vi "PositionCountTest.vi"() -> ()   [LabVIEW 2015]
uses:
  QuadEnc/QuadEnc.lvlib
panel:
  out "RevPosition 2":i32
  out "AbsPosition 2":i32
  in  "number of iterations":i32=20
  in  "spoofed tick rate":u32=20
  in  "spoofed ticks per rev":u32=10
  out "RevPosition":i32=999
  out "AbsPosition":i32=1999
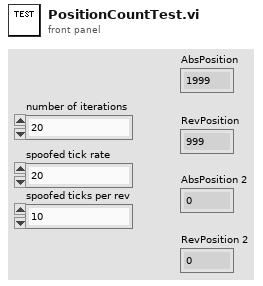
[diagram p1: front panel]
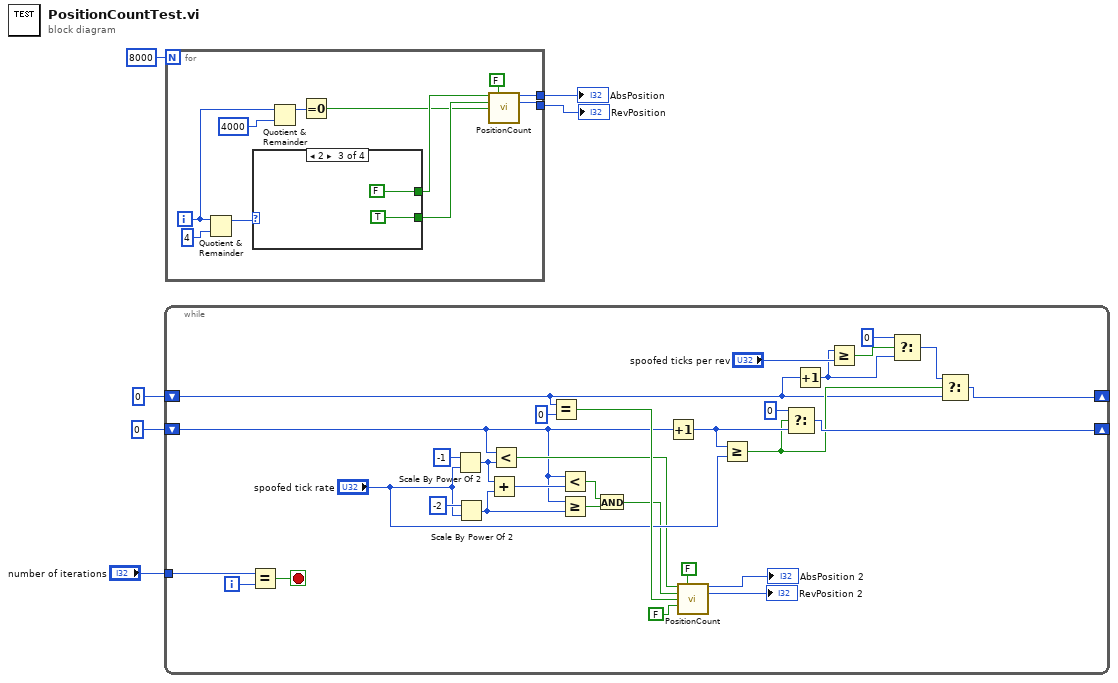
[diagram p0: block diagram]
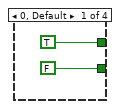
[diagram p2: hidden frame]
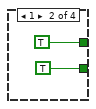
[diagram p3: hidden frame]
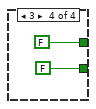
[diagram p4: hidden frame]
diagram:
  n1 = while {
    shift-right: [w26] -> _
    shift-left: u32 0 -> [w11]
    shift-right: [w25] -> _
    shift-left: u32 0 -> [w10]
    tunnel: "number of iterations" -> [w18]
    i -> [w16]
    stop <- w24 stop-if-true
    n2 = Equal?(x=w18, y=w16) -> (x = y?=w24:bool)
    n3 = Scale By Power Of 2(n=i16 -1, x="spoofed tick rate") -> (x*2^n=w34:u32)
    n4 = Scale By Power Of 2(n=i16 -2, x="spoofed tick rate") -> (x*2^n=w33:u32)
    n5 = Add(x=w34, y=w33) -> (x+y=w32:u32)
    n6 = Less?(x=w11, y=w34) -> (x < y?=w13:bool)
    n7 = Equal?(x=w10, y=u32 0) -> (x = y?=w19:bool)
    n8 = Less?(x=w11, y=w32) -> (x < y?=w31:bool)
    n9 = Greater Or Equal?(x=w11, y=w33) -> (x >= y?=w30:bool)
    n10 = And(x=w31, y=w30) -> (x .and. y?=w14:bool)
    n11 = Increment(x=w11) -> (x+1=w27:u32)
    n12 = call "PositionCount.vi"("A"=w13, "ReversePolarity"=FALSE, "B"=w14, "Z"=w19, "reset"=FALSE) -> ("AbsPosition"=→"AbsPosition 2":i32, "RevPosition"=→"RevPosition 2":i32)  [unwired: 8 in, 1 out]
    n13 = Greater Or Equal?(x=w27, y="spoofed tick rate") -> (x >= y?=w12:bool)
    n14 = Select(t=u32 0, s=w12, f=w27) -> (s? t:f=w26:u32)
    n15 = Increment(x=w10) -> (x+1=w8:u32)
    n16 = Greater Or Equal?(x=w8, y="spoofed ticks per rev") -> (x >= y?=w9:bool)
    n17 = Select(t=u32 0 ("s? t:f"), s=w9, f=w8) -> (s? t:f=w7:u32)
    n18 = Select(t=w7, s=w12, f=w10) -> (s? t:f=w25:u32)
  }
  n19 = for {
    N: 8000 -> [_]
    tunnel: [w43] -> w6
    tunnel: [w42] -> w5
    i -> [w41]
    n20 = Quotient & Remainder(x=w41, y=4) -> (x-y*floor(x/y)=w46:i32)  [unwired: 1 out]
    n21 = case shown="2" w46 {
      tunnel: [TRUE TRUE FALSE FALSE] -> w45
      tunnel: [FALSE TRUE TRUE FALSE] -> w44
      frame 0, Default {
      }
      frame 1 {
      }
      frame 2 {
      }
      frame 3 {
      }
    }
    n22 = Quotient & Remainder(x=w41, y=4000) -> (x-y*floor(x/y)=w39:i32)  [unwired: 1 out]
    n23 = Equal To 0?(x=w39) -> (x = 0?=w38:bool)
    n24 = call "PositionCount.vi"("A"=w45, "ReversePolarity"=FALSE, "B"=w44, "Z"=w38) -> ("AbsPosition"=w43:i32, "RevPosition"=w42:i32)  [unwired: 9 in, 1 out]
  }
  "AbsPosition" <- w6
  "RevPosition" <- w5
